vi "Rename Alias.vi"(6 "Remote Timeout (300,000 ms)":u32=300000, 7 "Update Dependencies (T)":bool=TRUE, 8 "error in (no error)":errorcluster, 9 "Overwrite Conflict (F)":bool, 10 "New Name":string, 11 "Resource in":refnum<k20>) -> (0 "error out":errorcluster, 1 "Overwritten Resource":refnum<k20>, 2 "Name Already Existed":bool, 3 "Resource out":refnum<k20>)   [LabVIEW 2017, in "nisyscfg.lvlib"]
doc: "Changes the display name of a resource."
uses:
  <vilib>/nisyscfg/nisyscfg.lvlib
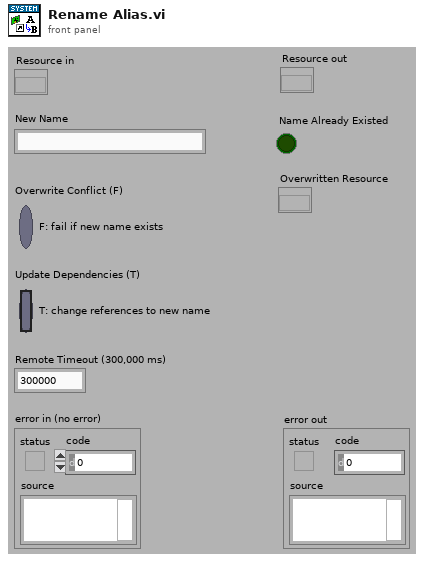
[diagram p1: front panel]
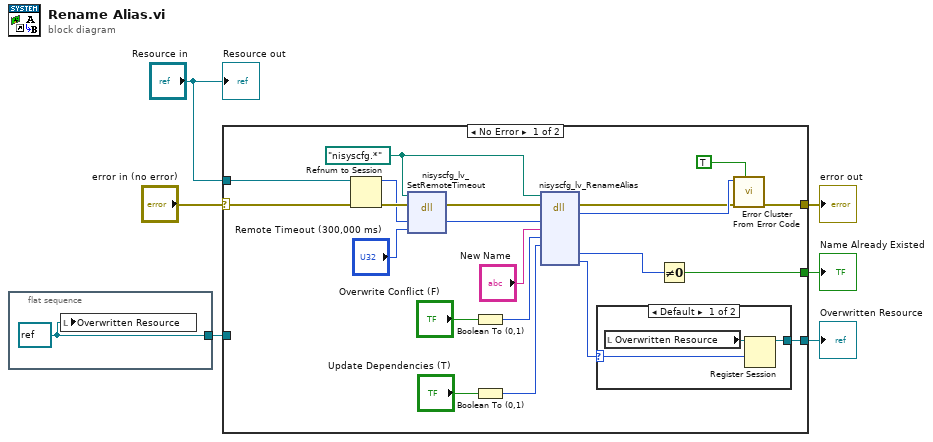
[diagram p0: block diagram]
diagram:
  n1 = flat-sequence {
    tunnel: [w7] -> w1
    frame #0 {
      w7 = refnum<k20> refnum ("filter in")
      n2 = local write "Overwritten Resource"(w7) -> ()
    }
  }
  n3 = case shown="No Error" "error in (no error)" {
    selector: "error in (no error)" -> [w17 w32]
    tunnel: [w26 w32] -> w6
    tunnel: "Resource in" -> [w16 _]
    tunnel: [w10 _] -> w3
    tunnel: [w8 _] -> w2
    tunnel: w1 -> [_ _]
    frame No Error {
      w15 = path "nisyscfg.*" ("path in")
      n4 = Refnum to Session(4:w17, 7:w16) -> (0:w25:errorcluster, 3:w23:u64)
      n5 = dll-call lib="nisyscfg.*" fn="nisyscfg_lv_SetRemoteTimeout" label="SetRemoteTimeout"(path in=w15, error in=w25, "item"=w23, "connectTimeout"="Remote Timeout (300,000 ms)") -> (error out=w24:errorcluster, "item"=w21:u64)  [unwired: 1 in, 3 out]
      n6 = Boolean To (0,1)(Boolean="Overwrite Conflict (F)") -> (0, 1=w12:i16)
      n7 = Boolean To (0,1)(Boolean="Update Dependencies (T)") -> (0, 1=w18:i16)
      n8 = dll-call lib="nisyscfg.*" fn="nisyscfg_lv_RenameAlias" label="RenameAlias"(path in=w15, error in=w24, "item"=w21, "newName"="New Name", "overwriteIfExists"=w12, "updateDependencies"=w18) -> (error out=w27:errorcluster, "status"=w28:i32, "nameExisted"=w11:u8, "otherResource"=w9:u64)  [unwired: 5 in, 3 out]
      n9 = case shown="Default" w9 {
        selector: w9 -> [w31 _]
        tunnel: [w30 _] -> w8
        frame Default {
          n10 = local read "Overwritten Resource"() -> (w29:refnum<k20>)
          n11 = Register Session(9:w31, 11:w29) -> (3:w30:refnum<k20>)  [unwired: 3 in, 1 out]
        }
        frame 0 {
        }
      }
      n12 = Not Equal To 0?(x=w11) -> (x != 0?=w10:bool)
      n13 = call <vilib>:"Error Cluster From Error Code.vi"("show call chain? (False)"=TRUE, "error in (no error)"=w27, "error code (0)"=w28) -> ("error out"=w26:errorcluster)  [unwired: 6 out]
    }
    frame Error {
    }
  }
  "error out" <- w6
  "Overwritten Resource" <- w2
  "Name Already Existed" <- w3
  "Resource out" <- "Resource in"
